vi "RP Write Command TCP.vi"(4 "bytes to read":i32=-1, 5 "Payload data":string, 6 "timeout ms (25000)":i32=1000, 7 "Config offset":u64, 8 "Error In":errorcluster, 9 "Command payload":u64 format="%x", 10 "Command number":T1, 11 "connection ID":refnum<k5>) -> (0 "Error Out":errorcluster, 1 "bytes written":i32, 2 "data out":string, 3 "connection ID out":refnum<k5>)   [LabVIEW 2024]
uses:
  RP Command.ctl
panel:
  out "x .or. y?":u64 format="%x"
  out "x << y":u64 format="%x"
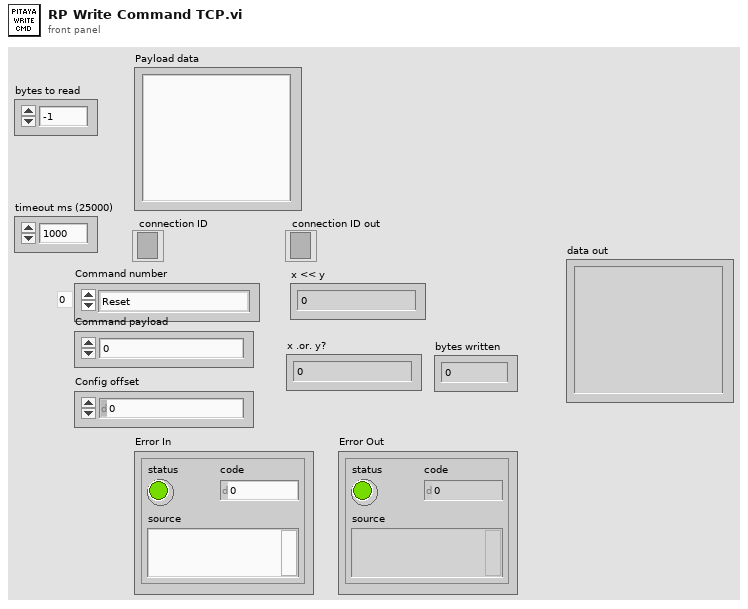
[diagram p1: front panel]
types:
  T1 = typedef "RP Command.ctl" = enum16{"Reset", "Read IDN", "Stop server", "Get status", "Get temperature", "Connect client", "Arm", "Software trigger", "Get whole buffer", "Get chunk", "System call", "Get config", "Set config", "Recieve data", "Recieve Calibartion", "Transmit data"}
  T2 = enum16{"big-endian, network order", "native, host order", "little-endian"}
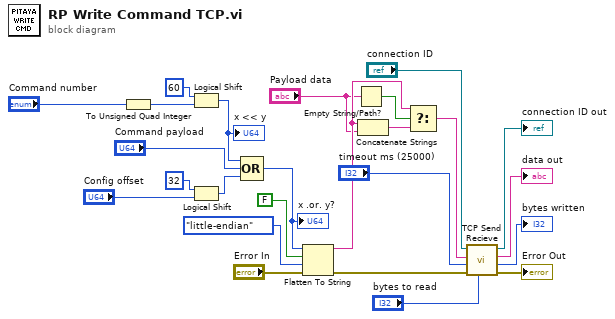
[diagram p0: block diagram]
diagram:
  n1 = To Unsigned Quad Integer(1:"Command number") -> (0:w17:u64)
  n2 = Logical Shift(y=i16 60, x=w17) -> (x << y=w23:u64)
  "x << y" <- w23
  n3 = Logical Shift(y=i16 32, x="Config offset") -> (x << y=w14:u64)
  n4 = Compound Arithmetic op=OR(w23, "Command payload", w14) -> (w18:u64)
  "x .or. y?" <- w18
  n5 = Flatten To String(anything=w18, prepend array or string size? (T)=FALSE, byte order (0:big-endian, network order)=T2."little-endian", error in (no error)="Error In") -> (data string=w4:string, error out=w12:errorcluster)  [unwired: 1 out]
  n6 = Empty String/Path?(string/path="Payload data") -> (empty?=w5:bool)
  n7 = Concatenate Strings(w4, "Payload data") -> (w2:string)
  n8 = Select(t=w4, s=w5, f=w2) -> (s? t:f=w1:string)
  n9 = call "TCP Send Recieve.vi"("bytes to read"="bytes to read", "Error In"=w12, "timeout ms (25000)"="timeout ms (25000)", "data in"=w1, "connection ID"="connection ID") -> ("Error Out"=→"Error Out":errorcluster, "bytes written"=→"bytes written":i32, "data out"=→"data out":string, "connection ID out"=→"connection ID out":refnum<k5>)  [unwired: 3 in]
